vi "Get Spectrum.vi"(8 "error in (no error)":errorcluster, 10 "Channel":u8, 11 "Spectrometer Driver in":refnum<class "Spectrometer Driver.lvclass">) -> (0 "error out":errorcluster, 2 "Spectrum Graph":cluster{dbl[], "Spectrum, db":dbl[]}[](graph), 3 "Spectrometer Driver out":refnum<class "Spectrometer Driver.lvclass">)   [LabVIEW 2016, in "Spectrometer Driver.lvclass"]
uses:
  Spectrometer Driver.lvclass
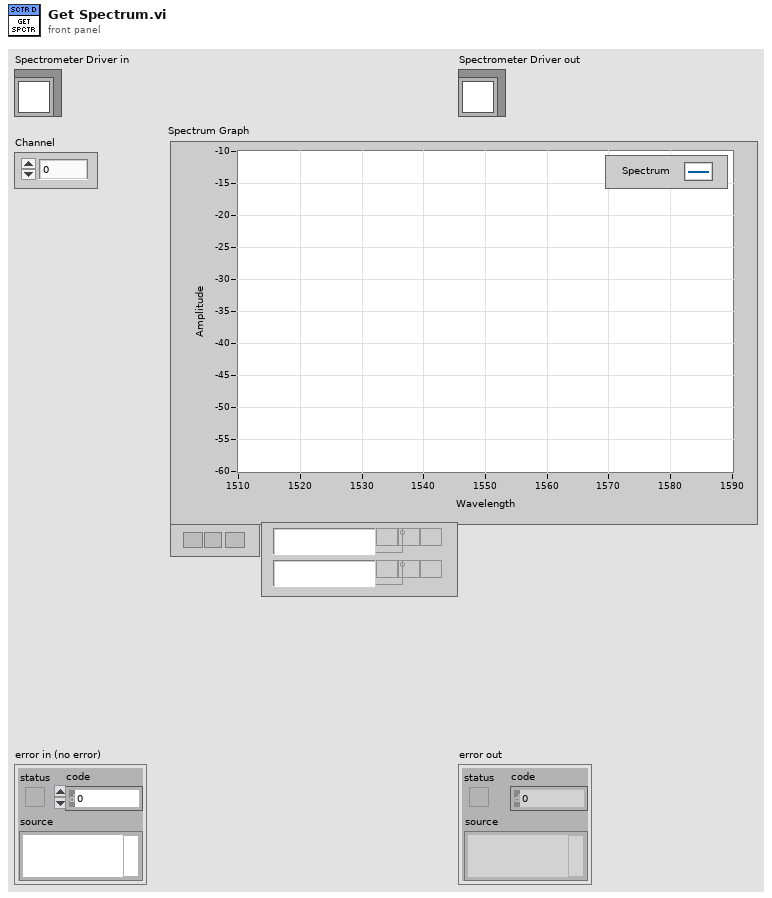
[diagram p1: front panel]
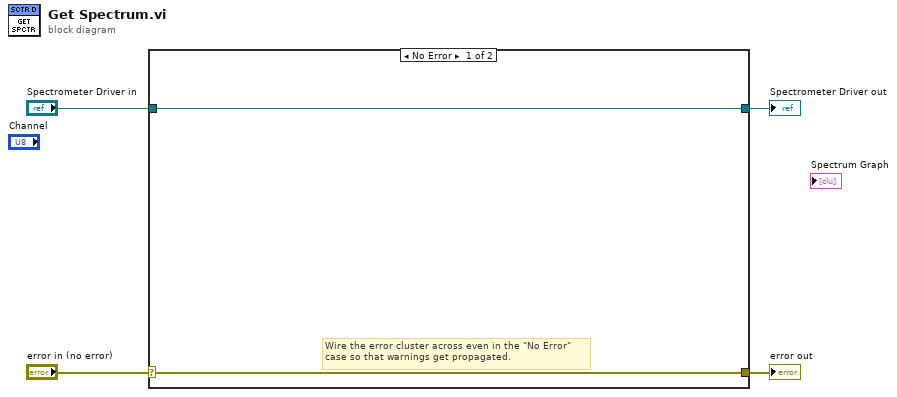
[diagram p0: block diagram]
diagram:
  n1 = case shown="No Error" "error in (no error)" {
    selector: "error in (no error)" -> [w5 w8]
    tunnel: [w5 w8] -> w3
    tunnel: [w6 w7] -> w1
    tunnel: "Spectrometer Driver in" -> [w6 w7]
    frame No Error {
      # "Wire the error cluster across even in the \"No Error\"\ncase so that warnings get propagated."
    }
    frame Error {
    }
  }
  "error out" <- w3
  "Spectrometer Driver out" <- w1
